vi "GetAttributeViString_ACP_SE_TOI.vi"(7 "AttributeValueBufferSize":i32=256 caption="AttributeValueBufferSize (256)", 8 "error in (no error)":errorcluster {"code" format="%.0x"}, 9 "AttributeID":u32(ring)=1150150 items=["SA_ACP_DISPLAY_TEXT"=1150150], 11 "instrument handle":refnum<k15>) -> (0 "error out":errorcluster {"code" format="%.0x"}, 2 "AttributeValue":string, 3 "instrument handle out":refnum<k15>)   [LabVIEW 2009, in "Keysight XSAn.lvlib"]
doc: "Gets a String attribute from the instrument driver.\nThe following Attributes are supported:\n\nSA_ACP_DISPLAY_TEXT"
uses:
  <instrlib>/Keysight XSAn/Keysight XSAn.lvlib
  AgXSAn.dll
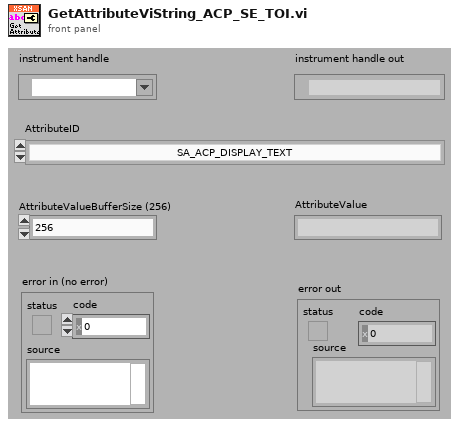
[diagram p1: front panel]
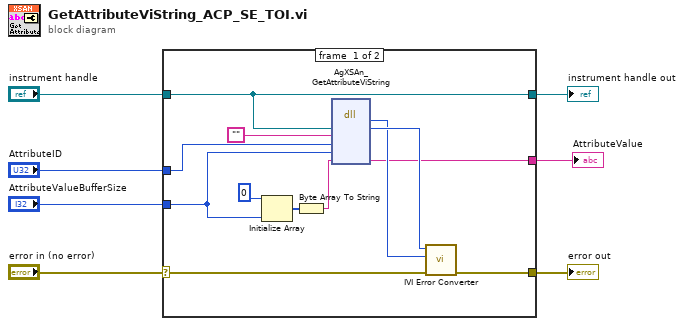
[diagram p0: block diagram]
diagram:
  n1 = case shown="No Error" "error in (no error)" {
    selector: "error in (no error)" -> [w17 w21]
    tunnel: [w16 w21] -> w7
    tunnel: "instrument handle" -> [w10 w20]
    tunnel: "AttributeID" -> [w15 _]
    tunnel: "AttributeValueBufferSize" -> [w9 _]
    tunnel: [w11 _] -> w2
    tunnel: [w10 w20] -> w1
    frame #0 {
      n2 = Initialize Array(u8 0 ("element"), w9) -> (w13:u8[])
      n3 = Byte Array To String(unsigned byte array=w13) -> (string=w14:string)
      n4 = dll-call lib="AgXSAn**.dll" fn="AgXSAn_GetAttributeViString"("Vi"=w10, "RepCapIdentifier"="", "AttributeID"=w15, "AttributeValueBufferSize"=w9, "AttributeValue"=w14) -> ("return type"=w18:i32, "Vi"=w19:u32, "AttributeValue"=w11:string)  [unwired: 6 in, 2 out]
      n5 = call <instrlib>:"IVI Error Converter.vi"("error in (no error)"=w17, "IVI error code (0)"=w18, "instrument handle"=w19) -> ("error out"=w16:errorcluster)  [unwired: 7 in, 1 out]
    }
    frame #1 {
    }
  }
  "error out" <- w7
  "instrument handle out" <- w1
  "AttributeValue" <- w2
